vi "Parse Request.vi"(8 "error in (no error)":errorcluster, 10 "JSON Request":string, 11 "JSON-RPC in":refnum<class "JSON-RPC.lvclass">) -> (0 "error out":errorcluster, 1 "Params":variant[](array[variant]), 2 "Methods":string[](array[string]), 3 "JSON-RPC out":refnum<class "JSON-RPC.lvclass">)   [LabVIEW 2019, in "JSON-RPC.lvclass"]
uses:
  JSON-RPC.lvclass
  Response/Response.lvclass
  JSON-RPC.lvclass/JSON-RPC.ctl
  lv-venv/lv.lib/vi.lib/addons/_JKI.lib/Serialization/JSON/JKI JSON Serialization.lvlib
  <vilib>/Utility/Data Type/NI_Data Type.lvlib
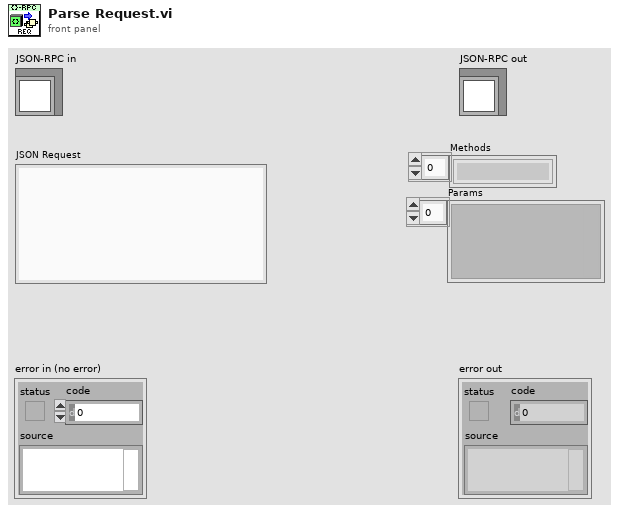
[diagram p1: front panel]
types:
  T1 = typedef "NI_Data Type.lvlib/Data Type.ctl" = enum8{"Invalid Type", "Void", "I8", "I16", "I32", "I64", "U8", "U16", "U32", "U64", "Single Float", "Double Float", "Extended Float", "Single Complex", "Double Complex", "Extended Complex", "Enum U8", "Enum U16", "Enum U32", "Enum U64", "Single Float With Unit", "Double Float With Unit", "Extended Float With Unit", "Single Complex with Unit", "Double Complex with Unit", "Extended Complex with Unit", "Boolean", "String", "Path", "Picture", "Tag", "Array", "Cluster", "Variant", "LV Variant", "Waveform", "Timestamp", "Digital Waveform", "Digital Data", "ExpressData", "Refnum", "External Data", "VI", "Poly VI", "LabVIEW Class Instance", "Fixed Point", "Set Collection", "Map Collection"}
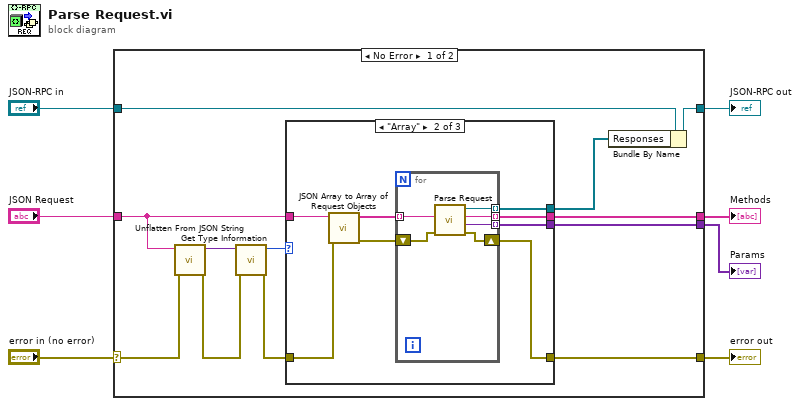
[diagram p0: block diagram]
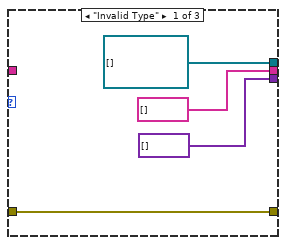
[diagram p2: hidden frame]
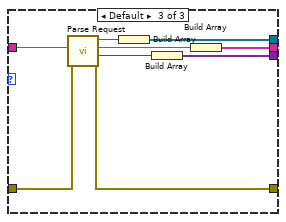
[diagram p3: hidden frame]
diagram:
  n1 = case shown="No Error" "error in (no error)" {
    selector: "error in (no error)" -> [w19 w48]
    tunnel: [w13 w48] -> w6
    tunnel: [w17 w47] -> w4
    tunnel: "JSON-RPC in" -> [w18 w47]
    tunnel: "JSON Request" -> [w10 _]
    tunnel: [w9 _] -> w1
    tunnel: [w8 _] -> w2
    frame No Error {
      n2 = call "Unflatten From JSON String.vi"("error in (no error)"=w19, "JSON String"=w10) -> ("error out"=w15:errorcluster, "Variant"=w14:variant)  [unwired: 8 in]
      n3 = call <vilib>:"Get Type Information.vi"("error in (no error)"=w15, "variant"=w14) -> ("error out"=w11:errorcluster, "type"=w16:T1)  [unwired: 5 in, 3 out]
      n4 = case shown="\"Array\"" w16 {
        tunnel: [refnum<class "Response.lvclass">[] [] w31 w44] -> w12
        tunnel: w11 -> [w23 w27 w43]
        tunnel: [w23 w30 w45] -> w13
        tunnel: w10 -> [_ w28 w42]
        tunnel: [string[] [] w25 w40] -> w8
        tunnel: [variant[] [] w24 w38] -> w9
        frame "Invalid Type" {
        }
        frame "Array" {
          n5 = call "JSON Array to Array of Request Objects.vi"("error in (no error)"=w27, "JSON Array"=w28) -> ("error out"=w29:errorcluster, "Request Objects"=w26:string[])  [unwired: 8 in]
          n6 = for {
            tunnel: [w37] -> w31 mode=indexing
            shift-right: [w35] -> w30
            shift-left: w29 -> [w36]
            tunnel: w26 -> [w34] mode=indexing
            tunnel: [w33] -> w25 mode=indexing
            tunnel: [w32] -> w24 mode=indexing
            n7 = call "Parse Request.vi"("error in (no error)"=w36, "JSON Request"=w34) -> ("error out"=w35:errorcluster, "params"=w32:variant, "method"=w33:string, "Response out"=w37:refnum<class "Response.lvclass">)  [unwired: 6 in]
          }
        }
        frame Default {
          n8 = call "Parse Request.vi"("error in (no error)"=w43, "JSON Request"=w42) -> ("error out"=w45:errorcluster, "params"=w39:variant, "method"=w41:string, "Response out"=w46:refnum<class "Response.lvclass">)  [unwired: 6 in]
          n9 = Build Array(w46) -> (w44:refnum<class "Response.lvclass">[])
          n10 = Build Array(w39) -> (w38:variant[])
          n11 = Build Array(w41) -> (w40:string[])
        }
      }
      n12 = Bundle By Name(cluster=w18, "Responses"=w12) -> (w17:refnum<class "JSON-RPC.lvclass">)
    }
    frame Error {
    }
  }
  "error out" <- w6
  "JSON-RPC out" <- w4
  "Methods" <- w2
  "Params" <- w1
